vi "TubingCompensation.vi"(7 "NyquistLimitedCoefficients":dbl[](array[numeric]), 9 "NyquistLimitedPhase":dbl[](array[numeric]), 10 "mutedData":dbl[](array[numeric]), 11 "SamplingFreq":dbl) -> (1 "boostedDataNaNdEnds":dbl[](array[numeric]), 2 "boostedData":dbl[](array[numeric]))   [LabVIEW 2016]
uses:
  <vilib>/Analysis/NI_AALBase.lvlib
panel:
  in  "EndKiller(pts)":i32=3
  out "SDincrease(%)":dbl format="%.1f"
  out "Waveform Graph":dbl[][](graph)
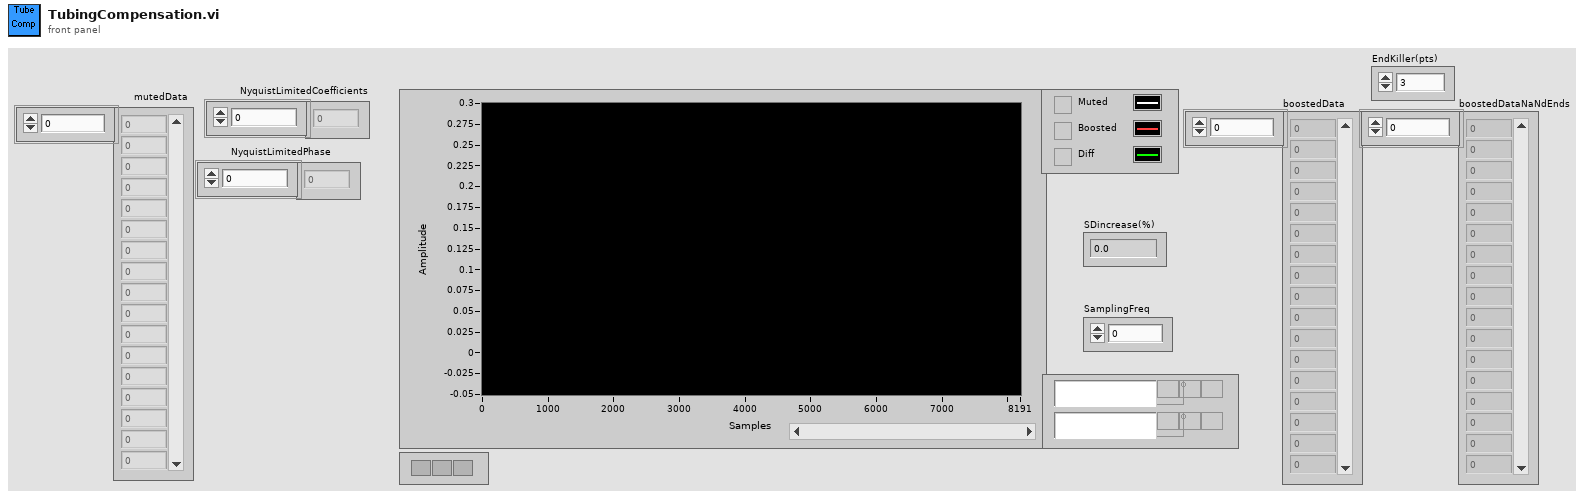
[diagram p1: front panel]
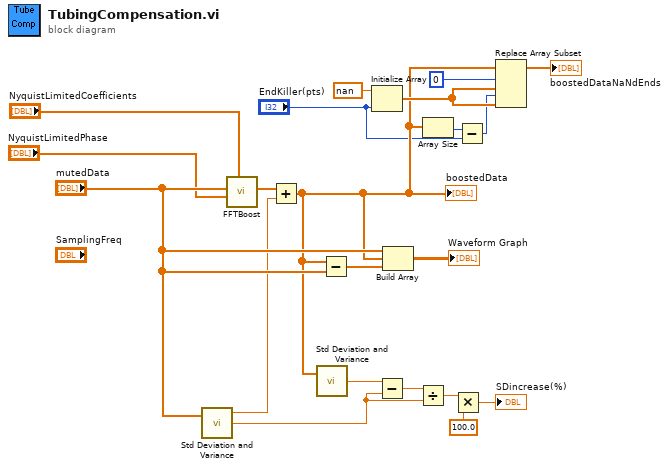
[diagram p0: block diagram]
diagram:
  n1 = call <vilib>:"Std Deviation and Variance.vi"("X"="mutedData") -> ("mean"=w11:dbl, "standard deviation"=w15:dbl)  [unwired: 1 in, 1 out]
  n2 = call "FFTBoost.vi"("CompensationCoefficients"="NyquistLimitedCoefficients", "PhaseCorrection"="NyquistLimitedPhase", "mutedData"="mutedData") -> ("boostedData"=w18:dbl[])  [unwired: 1 in, 7 out]
  n3 = Add(x=w18, y=w11) -> (x+y=w3:dbl[])
  "boostedData" <- w3
  n4 = call <vilib>:"Std Deviation and Variance.vi"("X"=w3) -> ("standard deviation"=w17:dbl)  [unwired: 1 in, 2 out]
  n5 = Subtract(x=w3, y="mutedData") -> (x-y=w20:dbl[])
  n6 = Initialize Array(nan ("element"), "EndKiller(pts)") -> (w6:dbl[])
  n7 = Subtract(x=w17, y=w15) -> (x-y=w16:dbl)
  n8 = Build Array("mutedData", w3, w20) -> (→"Waveform Graph":dbl[][])
  n9 = Divide(x=w16, y=w15) -> (x/y=w14:dbl)
  n10 = Array Size(array=w3) -> (size(s)=w5:i32)
  n11 = Multiply(x=w14, y=100.0) -> (x*y=→"SDincrease(%)":dbl)
  n12 = Subtract(x=w5, y="EndKiller(pts)") -> (x-y=w4:i32)
  n13 = Replace Array Subset(array=w3, new element #1=w6, index #1=0 ("index"), new element #2=w6, index #2=w4) -> (→"boostedDataNaNdEnds":dbl[])
